vi "Files_Test_Matlab.vi"() -> ()   [LabVIEW 2026]
panel:
  in  "Temps de pause (s)":dbl
  out "All 2":u32
  out "All":u32
  out "End":u32
  out "Function":dbl
  out "Start":u32
  out "sortie d'erreur":errorcluster
  in  "entrée d'erreur (pas d'erreur)":errorcluster
  in  "Repetitions":i32
  out "Tableau":dbl[](array[numeric])
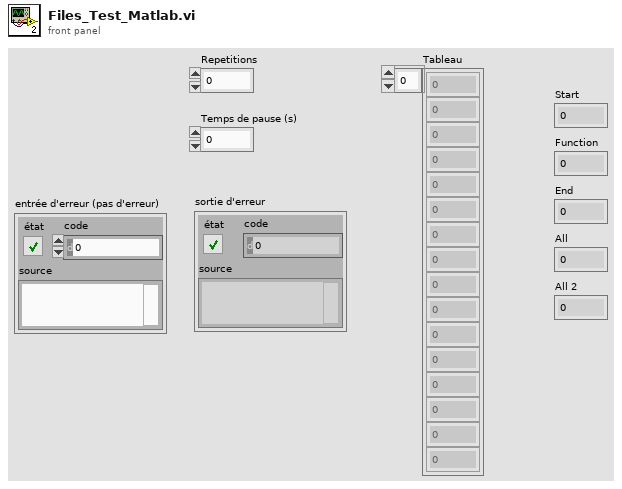
[diagram p1: front panel]
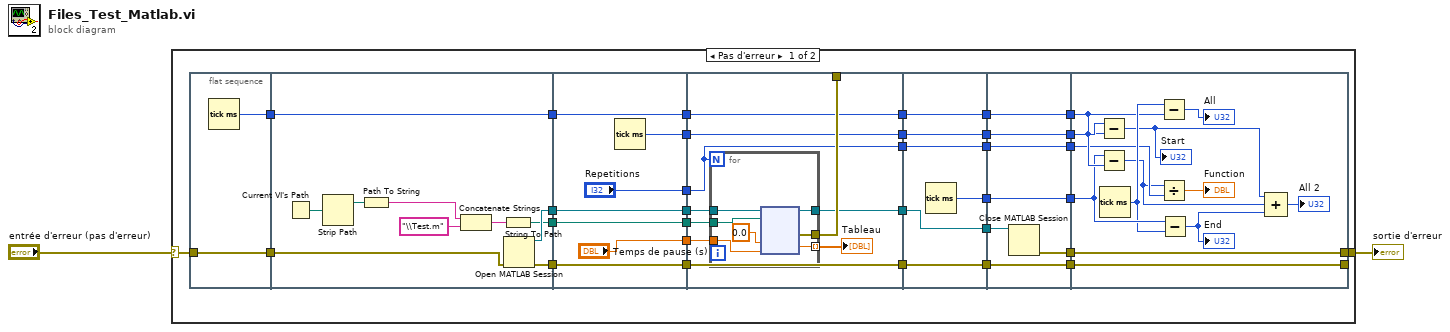
[diagram p0: block diagram]
diagram:
  n1 = case shown="Pas d'erreur" "entrée d'erreur (pas d'erreur)" {
    selector: "entrée d'erreur (pas d'erreur)" -> [w34 w97]
    tunnel: [w33 w97] -> w2
    frame No Error {
      n2 = flat-sequence {
        tunnel: w34 -> [w36]
        tunnel: [w36] -> w32
        tunnel: [w35] -> w19
        tunnel: [w46] -> w31
        tunnel: [w45] -> w30
        tunnel: [w39] -> w29
        tunnel: w32 -> [w38]
        tunnel: w19 -> [w37]
        tunnel: [w37] -> w18
        tunnel: w31 -> [w53]
        tunnel: [w53] -> w28
        tunnel: w30 -> [w52]
        tunnel: [w52] -> w27
        tunnel: w29 -> [w51]
        tunnel: [w51] -> w26
        tunnel: w18 -> [w50]
        tunnel: [w50] -> w17
        tunnel: [w49] -> w13
        tunnel: ["Repetitions"] -> w4
        tunnel: ["Temps de pause (s)"] -> w3
        tunnel: w28 -> [w60]
        tunnel: w27 -> [w63]
        tunnel: w26 -> [w58]
        tunnel: [w63] -> w23
        tunnel: [w62] -> _
        tunnel: [w59] -> w21
        tunnel: w17 -> [w57]
        tunnel: [w57] -> w16
        tunnel: w13 -> [w56]
        tunnel: [w56] -> w12
        tunnel: [w55] -> w7
        tunnel: w4 -> [w55]
        tunnel: w3 -> [w54]
        tunnel: w23 -> [w76]
        tunnel: [w76] -> w22
        tunnel: w21 -> [w75]
        tunnel: [w75] -> w20
        tunnel: w16 -> [w74]
        tunnel: [w74] -> w15
        tunnel: w12 -> [w73]
        tunnel: [w73] -> w11
        tunnel: [w72] -> w9
        tunnel: w7 -> [w71]
        tunnel: [w71] -> w6
        tunnel: w22 -> [w83]
        tunnel: w20 -> [w81]
        tunnel: [w83] -> w25
        tunnel: [w82] -> w24
        tunnel: w15 -> [w80]
        tunnel: [w80] -> w14
        tunnel: w11 -> [w79]
        tunnel: [w79] -> w10
        tunnel: w9 -> [w78]
        tunnel: [w78] -> w8
        tunnel: w6 -> [w77]
        tunnel: [w77] -> w5
        tunnel: [w95] -> w33
        tunnel: [w96] -> _
        tunnel: w25 -> [w96]
        tunnel: w24 -> [w95]
        tunnel: w14 -> [w91]
        tunnel: w10 -> [w94]
        tunnel: w8 -> [w93]
        tunnel: w5 -> [w89]
        frame #0 {
          n3 = Tick Count (ms)() -> (millisecond timer value=w35:u32)
        }
        frame #1 {
          n4 = Current VI's Path() -> (path=w42:path)
          n5 = Strip Path(path=w42) -> (stripped path=w41:path)  [unwired: 1 out]
          n6 = Path To String(path=w41) -> (string=w43:string)
          n7 = Concatenate Strings(w43, "\\Test.m" ("chaîne")) -> (w44:string)
          n8 = String To Path(string=w44) -> (path=w39:path)
          n9 = Open MATLAB Session(3:w38) -> (8:w46:refnum<k37>, 11:w45:errorcluster)  [unwired: 1 in]
        }
        frame #2 {
          n10 = Tick Count (ms)() -> (millisecond timer value=w49:u32)
        }
        frame #3 {
          n11 = for {
            N: w55 -> [_]
            tunnel: [w70] -> w59
            tunnel: [w69] -> w62
            tunnel: [w67] -> w61 mode=indexing
            tunnel: w60 -> [w66]
            tunnel: w58 -> [w65]
            tunnel: w54 -> [w64]
            n12 = node ("Appeler une fonction MATLAB")(w66, w65, 0.0, w64) -> (w70:refnum<k37>, w69:errorcluster, w67:dbl)  [unwired: 3 in, 2 out]
          }
          "Tableau" <- w61
        }
        frame #4 {
          n13 = Tick Count (ms)() -> (millisecond timer value=w72:u32)
        }
        frame #5 {
          n14 = Close MATLAB Session(0:w81) -> (11:w82:errorcluster)  [unwired: 1 in]
        }
        frame #6 {
          n15 = Subtract(x=w94, y=w91) -> (x-y=w87:u32)
          "Start" <- w87
          n16 = Subtract(x=w93, y=w94) -> (x-y=w86:u32)
          n17 = Tick Count (ms)() -> (millisecond timer value=w92:u32)
          n18 = Subtract(x=w92, y=w91) -> (x-y=→"All":u32)
          n19 = Divide(x=w86, y=w89) -> (x/y=→"Function":dbl)
          n20 = Subtract(x=w93, y=w92) -> (x-y=w85:u32)
          "End" <- w85
          n21 = Compound Arithmetic op=ADD(w87, w86, w85) -> (→"All 2":u32)
        }
      }
    }
    frame Error {
    }
  }
  "sortie d'erreur" <- w2
